vi "Detector.vi"(8 "error in (no error)":errorcluster, 10 "Signal":cdb[](array[numeric]), 11 "Lock-in Detector in":refnum<class "Lock-in Detector.lvclass">) -> (0 "error out":errorcluster, 2 "Signal out":cdb[](array[numeric]), 3 "Lock-in Detector out":refnum<class "Lock-in Detector.lvclass">)   [LabVIEW 2021, in "Lock-in Detector.lvclass"]
uses:
  Lock-in Detector.lvclass
  Lock-in Detector.lvclass/Lock-in Detector.ctl
  Read Decimation factor.vi
  <vilib>/Analysis/2dsp.llb/Decimate (continuous, CDB).vi
  <vilib>/Analysis/NI_AALPro.lvlib
panel:
  out "Sig-Ref":dbl[][](graph)
  out "Waveform Graph 2":dbl[](graph)
  out "Waveform Graph":dbl[](graph)
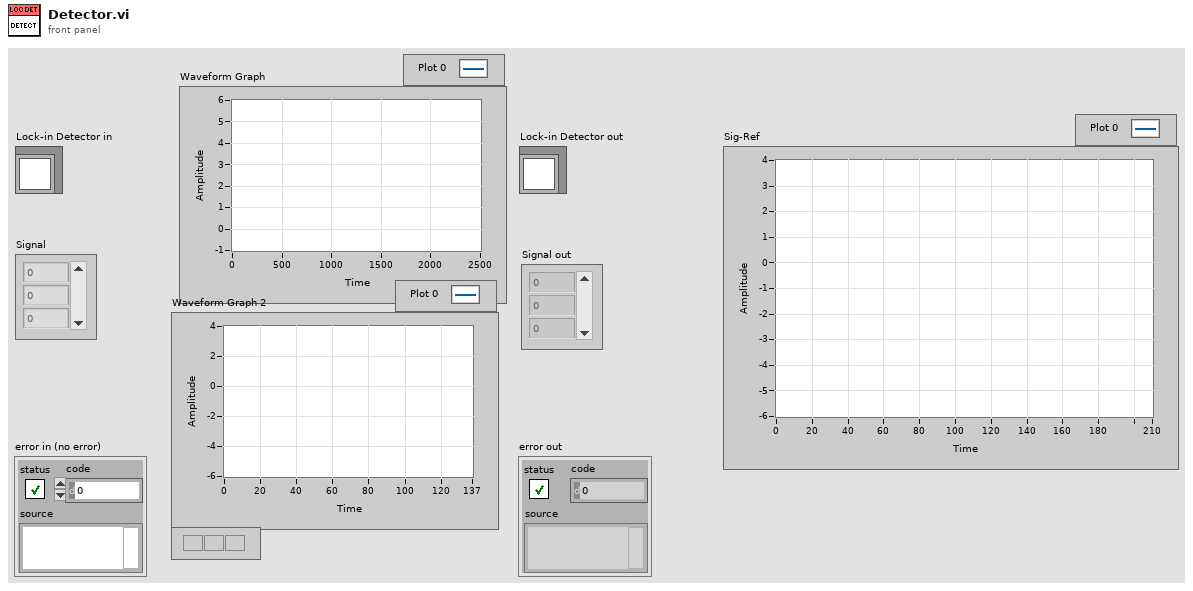
[diagram p1: front panel]
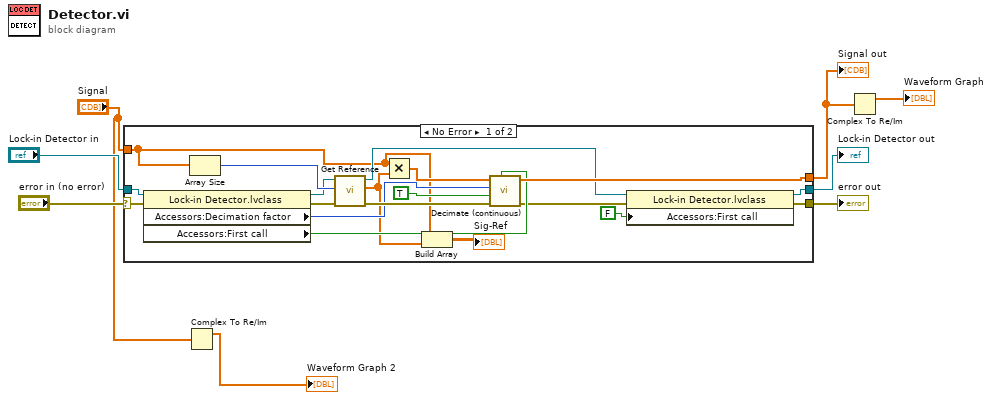
[diagram p0: block diagram]
diagram:
  n1 = case shown="No Error" "error in (no error)" {
    selector: "error in (no error)" -> [w20 w29]
    tunnel: [w12 w29] -> w7
    tunnel: [w15 w28] -> w5
    tunnel: "Lock-in Detector in" -> [w21 w28]
    tunnel: "Signal" -> [w11 _]
    tunnel: [w18 _] -> w4
    frame No Error {
      n2 = property class="Lock-in Detector.lvclass"(reference=w21, error in=w20) -> (reference out=w19:refnum<class "Lock-in Detector.lvclass">, error out=w26:errorcluster, "Accessors:Decimation factor"=w22:i32, "Accessors:First call"=w17:bool)
      n3 = Array Size(array=w11) -> (size(s)=w27:i32)
      n4 = call-dynamic "Get Reference.vi"("error in (no error)"=w26, "Samples"=w27, "Lock-in Detector in"=w19) -> ("error out"=w24:errorcluster, "Reference"=w10:cdb[], "Lock-in Detector out"=w14:refnum<class "Lock-in Detector.lvclass">)  [unwired: 6 in]
      n5 = Multiply(x=w11, y=w10) -> (x*y=w25:cdb[])
      n6 = Build Array(w11, w10) -> (→"Sig-Ref":cdb[][])
      n7 = call-poly <vilib>:"Decimate (continuous).vi"("reset"=w17, "error in (no error)"=w24, "averaging"=TRUE, "decimating factor"=w22, "X"=w25) -> ("error out"=w13:errorcluster, "Decimated Array"=w18:cdb[])  [unwired: 5 in]
      n8 = property class="Lock-in Detector.lvclass"(reference=w14, error in=w13, "Accessors:First call"=FALSE ("First call")) -> (reference out=w15:refnum<class "Lock-in Detector.lvclass">, error out=w12:errorcluster)
    }
    frame Error {
    }
  }
  "error out" <- w7
  "Lock-in Detector out" <- w5
  "Signal out" <- w4
  n9 = Complex To Re/Im(x + iy="Signal") -> (x=→"Waveform Graph 2":dbl[])  [unwired: 1 out]
  n10 = Complex To Re/Im(x + iy=w4) -> (x=→"Waveform Graph":dbl[])  [unwired: 1 out]
